vi "Auto_Routine_Deposit_Balance.vi"(8 "error in (no error)":errorcluster, 10 "Game Piece":T1, 11 "Position":T2=enum."Middle") -> (0 "error out":errorcluster)   [LabVIEW 2023]
uses:
  Arm/ArmPositionPreset.ctl
  Arm/ArmGamePiecePreset.ctl
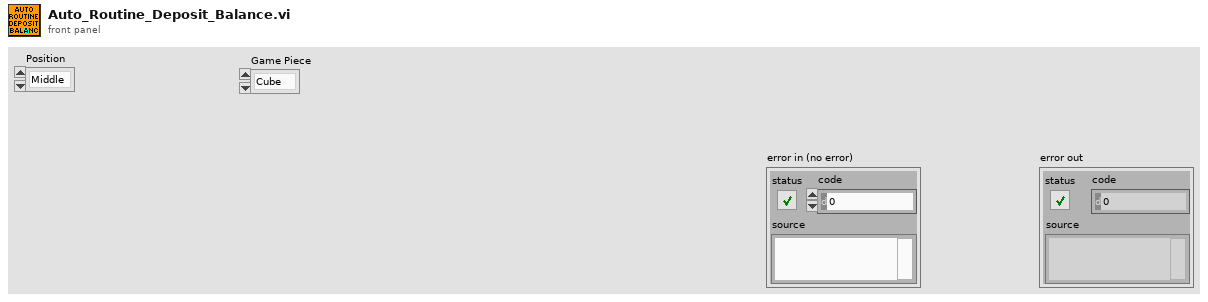
[diagram p1: front panel]
types:
  T1 = typedef "ArmGamePiecePreset.ctl" = enum16{"Cube", "Cone"}
  T2 = typedef "ArmPositionPreset.ctl" = enum16{"Upper", "Lower", "Middle", "Home", "Shelf", "Floor", "HalfFloor", "HalfHome"}
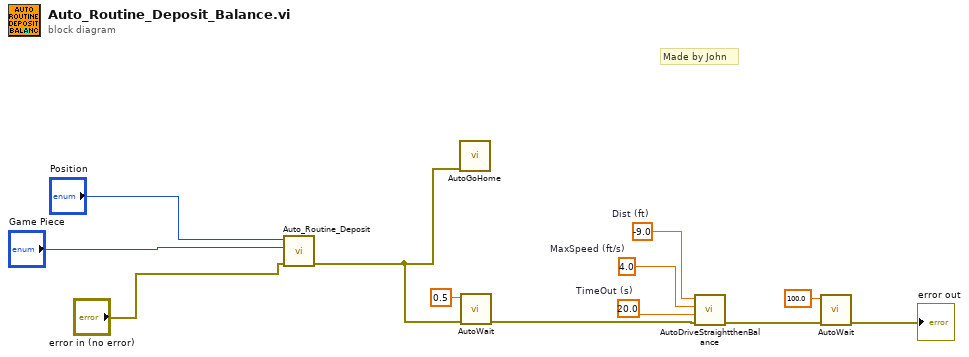
[diagram p0: block diagram]
diagram:
  w10 = 20.0  # TimeOut (s)
  w11 = 4.0  # MaxSpeed (ft/s)
  w12 = -9.0  # Dist (ft)
  # "Made by John"
  n1 = call "Auto_Routine_Deposit.vi"("error in (no error)"="error in (no error)", "Game Piece"="Game Piece", "Position"="Position") -> ("error out"=w5:errorcluster)  [unwired: 8 in]
  n2 = call "AutoGoHome.vi"("error in (no error)"=w5) -> ()  [unwired: 10 in, 1 out]
  n3 = call "AutoWait.vi"("error in (no error)"=w5, "TimeOut (s)"=0.5) -> ("error out"=w4:errorcluster)  [unwired: 9 in]
  n4 = call "AutoDriveStraightthenBalance.vi"("error in (no error)"=w4, "TimeOut (s)"=w10, "MaxSpeed (ft/s)"=w11, "Dist (ft)"=w12) -> ("error out"=w3:errorcluster)  [unwired: 7 in]
  n5 = call "AutoWait.vi"("error in (no error)"=w3, "TimeOut (s)"=100.0) -> ("error out"=→"error out":errorcluster)  [unwired: 9 in]
